vi "Main.vi"(7 "sweep rate, /min":dbl=0.2, 8 "sweep to:":dbl=4.0, 9 "sweep":T8(radio)=enum."2636a_smub") -> ()   [LabVIEW 2021] (continued)
                # "2182A 1 channel 2 measure (2182A_1_ch2)"
                n1376 = local read "2182A 1 ch2"() -> (w1691:bool)
                n1377 = property on="Figure_axis" class="Arr (strict)"() -> ("Value"=w1688:string[])  [unwired: 2 in, 2 out]
                n1378 = property on="data_caption" class="Str"() -> ("Value"=w1690:string)  [unwired: 2 in, 2 out]
                n1379 = case shown="True" w1691 {
                  tunnel: w1690 -> [w1693 w1699]
                  tunnel: [w1693 w1698] -> w1689
                  tunnel: w1688 -> [w1692 w1696]
                  tunnel: [w1692 w1694] -> w1687
                  frame False {
                    # "not measure 2182A 1 channel 2 (2182A_1_ch2)"
                  }
                  frame True {
                    w1695 = "2182A_1_ch2"
                    # "measure 2182A 1 channel 2 (2182A_1_ch2)"
                    n1380 = local read "2182A 1 addr"() -> (w1700:u8)
                    n1381 = Number To Decimal String(number=w1700) -> (decimal integer string=w1701:string)  [unwired: 1 in]
                    n1382 = GPIB Clear(3:w1701) -> ()  [unwired: 1 in, 2 out]
                    n1383 = Build Array (concatenate)(w1696, w1695) -> (w1694:string[])
                    n1384 = Concatenate Strings(w1699, w1695, "\t") -> (w1698:string)
                  }
                }
                n1385 = property on="Figure_axis" class="Arr (strict)"("Value"=w1687) -> ()  [unwired: 2 in, 2 out]
                n1386 = property on="data_caption" class="Str"("Value"=w1689) -> ()  [unwired: 2 in, 2 out]
              }
              frame #18 {
                # "2182A 2 channel 1 measure (2182A_2_ch1)"
                n1387 = local read "2182A 2 ch1"() -> (w1706:bool)
                n1388 = property on="Figure_axis" class="Arr (strict)"() -> ("Value"=w1703:string[])  [unwired: 2 in, 2 out]
                n1389 = property on="data_caption" class="Str"() -> ("Value"=w1705:string)  [unwired: 2 in, 2 out]
                n1390 = case shown="True" w1706 {
                  tunnel: w1705 -> [w1708 w1714]
                  tunnel: [w1708 w1713] -> w1704
                  tunnel: w1703 -> [w1707 w1711]
                  tunnel: [w1707 w1709] -> w1702
                  frame False {
                    # "not measure 2182A 2 channel 1 (2182A_2_ch1)"
                  }
                  frame True {
                    w1710 = "2182A_2_ch1"
                    # "measure 2182A 2 channel 1 (2182A_2_ch1)"
                    n1391 = local read "2182A 2 addr"() -> (w1715:u8)
                    n1392 = Number To Decimal String(number=w1715) -> (decimal integer string=w1716:string)  [unwired: 1 in]
                    n1393 = GPIB Clear(3:w1716) -> ()  [unwired: 1 in, 2 out]
                    n1394 = Build Array (concatenate)(w1711, w1710) -> (w1709:string[])
                    n1395 = Concatenate Strings(w1714, w1710, "\t") -> (w1713:string)
                  }
                }
                n1396 = property on="Figure_axis" class="Arr (strict)"("Value"=w1702) -> ()  [unwired: 2 in, 2 out]
                n1397 = property on="data_caption" class="Str"("Value"=w1704) -> ()  [unwired: 2 in, 2 out]
              }
              frame #19 {
                # "2182A 2 channel 2 measure (2182A_2_ch2)"
                n1398 = local read "2182A 2 ch2"() -> (w1721:bool)
                n1399 = property on="Figure_axis" class="Arr (strict)"() -> ("Value"=w1718:string[])  [unwired: 2 in, 2 out]
                n1400 = property on="data_caption" class="Str"() -> ("Value"=w1720:string)  [unwired: 2 in, 2 out]
                n1401 = case shown="True" w1721 {
                  tunnel: w1720 -> [w1723 w1729]
                  tunnel: [w1723 w1728] -> w1719
                  tunnel: w1718 -> [w1722 w1726]
                  tunnel: [w1722 w1724] -> w1717
                  frame False {
                    # "not measure 2182A 2 channel 2 (2182A_2_ch2)"
                  }
                  frame True {
                    w1725 = "2182A_2_ch2"
                    # "measure 2182A 2 channel 2 (2182A_2_ch2)"
                    n1402 = local read "2182A 2 addr"() -> (w1730:u8)
                    n1403 = Number To Decimal String(number=w1730) -> (decimal integer string=w1731:string)  [unwired: 1 in]
                    n1404 = GPIB Clear(3:w1731) -> ()  [unwired: 1 in, 2 out]
                    n1405 = Build Array (concatenate)(w1726, w1725) -> (w1724:string[])
                    n1406 = Concatenate Strings(w1729, w1725, "\t") -> (w1728:string)
                  }
                }
                n1407 = property on="Figure_axis" class="Arr (strict)"("Value"=w1717) -> ()  [unwired: 2 in, 2 out]
                n1408 = property on="data_caption" class="Str"("Value"=w1719) -> ()  [unwired: 2 in, 2 out]
              }
              frame #20 {
                # "2182A 3 channel 1 measure (2182A_3_ch1)"
                n1409 = local read "2182A 3 ch1"() -> (w1736:bool)
                n1410 = property on="Figure_axis" class="Arr (strict)"() -> ("Value"=w1733:string[])  [unwired: 2 in, 2 out]
                n1411 = property on="data_caption" class="Str"() -> ("Value"=w1735:string)  [unwired: 2 in, 2 out]
                n1412 = case shown="True" w1736 {
                  tunnel: w1735 -> [w1738 w1744]
                  tunnel: [w1738 w1743] -> w1734
                  tunnel: w1733 -> [w1737 w1741]
                  tunnel: [w1737 w1739] -> w1732
                  frame False {
                    # "not measure 2182A 3 channel 1 (2182A_3_ch1)"
                  }
                  frame True {
                    w1740 = "2182A_3_ch1"
                    # "measure 2182A 3 channel 1 (2182A_3_ch1)"
                    n1413 = local read "2182A 3 addr"() -> (w1745:u8)
                    n1414 = Number To Decimal String(number=w1745) -> (decimal integer string=w1746:string)  [unwired: 1 in]
                    n1415 = GPIB Clear(3:w1746) -> ()  [unwired: 1 in, 2 out]
                    n1416 = Build Array (concatenate)(w1741, w1740) -> (w1739:string[])
                    n1417 = Concatenate Strings(w1744, w1740, "\t") -> (w1743:string)
                  }
                }
                n1418 = property on="Figure_axis" class="Arr (strict)"("Value"=w1732) -> ()  [unwired: 2 in, 2 out]
                n1419 = property on="data_caption" class="Str"("Value"=w1734) -> ()  [unwired: 2 in, 2 out]
              }
              frame #21 {
                # "2182A 3 channel 2 measure (2182A_3_ch2)"
                n1420 = local read "2182A 3 ch2"() -> (w1751:bool)
                n1421 = property on="Figure_axis" class="Arr (strict)"() -> ("Value"=w1748:string[])  [unwired: 2 in, 2 out]
                n1422 = property on="data_caption" class="Str"() -> ("Value"=w1750:string)  [unwired: 2 in, 2 out]
                n1423 = case shown="False" w1751 {
                  tunnel: w1750 -> [w1753 w1759]
                  tunnel: [w1753 w1758] -> w1749
                  tunnel: w1748 -> [w1752 w1756]
                  tunnel: [w1752 w1754] -> w1747
                  frame False {
                    # "not measure 2182A 3 channel 2 (2182A_3_ch2)"
                  }
                  frame True {
                    w1755 = "2182A_3_ch2"
                    # "measure 2182A 3 channel 2 (2182A_3_ch2)"
                    n1424 = local read "2182A 3 addr"() -> (w1760:u8)
                    n1425 = Number To Decimal String(number=w1760) -> (decimal integer string=w1761:string)  [unwired: 1 in]
                    n1426 = GPIB Clear(3:w1761) -> ()  [unwired: 1 in, 2 out]
                    n1427 = Build Array (concatenate)(w1756, w1755) -> (w1754:string[])
                    n1428 = Concatenate Strings(w1759, w1755, "\t") -> (w1758:string)
                  }
                }
                n1429 = property on="Figure_axis" class="Arr (strict)"("Value"=w1747) -> ()  [unwired: 2 in, 2 out]
                n1430 = property on="data_caption" class="Str"("Value"=w1749) -> ()  [unwired: 2 in, 2 out]
              }
              frame #22 {
                # "2182A 4 channel 1 measure (2182A_4_ch1)"
                n1431 = local read "2182A 4 ch1"() -> (w1766:bool)
                n1432 = property on="Figure_axis" class="Arr (strict)"() -> ("Value"=w1763:string[])  [unwired: 2 in, 2 out]
                n1433 = property on="data_caption" class="Str"() -> ("Value"=w1765:string)  [unwired: 2 in, 2 out]
                n1434 = case shown="True" w1766 {
                  tunnel: w1765 -> [w1768 w1774]
                  tunnel: [w1768 w1773] -> w1764
                  tunnel: w1763 -> [w1767 w1771]
                  tunnel: [w1767 w1769] -> w1762
                  frame False {
                    # "not measure 2182A 4 channel 1 (2182A_4_ch1)"
                  }
                  frame True {
                    w1770 = "2182A_4_ch1"
                    # "measure 2182A 4 channel 1 (2182A_4_ch1)"
                    n1435 = local read "2182A 4 addr"() -> (w1775:u8)
                    n1436 = Number To Decimal String(number=w1775) -> (decimal integer string=w1776:string)  [unwired: 1 in]
                    n1437 = GPIB Clear(3:w1776) -> ()  [unwired: 1 in, 2 out]
                    n1438 = Build Array (concatenate)(w1771, w1770) -> (w1769:string[])
                    n1439 = Concatenate Strings(w1774, w1770, "\t") -> (w1773:string)
                  }
                }
                n1440 = property on="Figure_axis" class="Arr (strict)"("Value"=w1762) -> ()  [unwired: 2 in, 2 out]
                n1441 = property on="data_caption" class="Str"("Value"=w1764) -> ()  [unwired: 2 in, 2 out]
              }
              frame #23 {
                # "2182A 4 channel 2 measure (2182A_4_ch2)"
                n1442 = local read "2182A 4 ch2"() -> (w1781:bool)
                n1443 = property on="Figure_axis" class="Arr (strict)"() -> ("Value"=w1778:string[])  [unwired: 2 in, 2 out]
                n1444 = property on="data_caption" class="Str"() -> ("Value"=w1780:string)  [unwired: 2 in, 2 out]
                n1445 = case shown="True" w1781 {
                  tunnel: w1780 -> [w1783 w1789]
                  tunnel: [w1783 w1788] -> w1779
                  tunnel: w1778 -> [w1782 w1786]
                  tunnel: [w1782 w1784] -> w1777
                  frame False {
                    # "not measure 2182A 4 channel 2 (2182A_4_ch2)"
                  }
                  frame True {
                    w1785 = "2182A_4_ch2"
                    # "measure 2182A 4 channel 2 (2182A_4_ch2)"
                    n1446 = local read "2182A 4 addr"() -> (w1790:u8)
                    n1447 = Number To Decimal String(number=w1790) -> (decimal integer string=w1791:string)  [unwired: 1 in]
                    n1448 = GPIB Clear(3:w1791) -> ()  [unwired: 1 in, 2 out]
                    n1449 = Build Array (concatenate)(w1786, w1785) -> (w1784:string[])
                    n1450 = Concatenate Strings(w1789, w1785, "\t") -> (w1788:string)
                  }
                }
                n1451 = property on="Figure_axis" class="Arr (strict)"("Value"=w1777) -> ()  [unwired: 2 in, 2 out]
                n1452 = property on="data_caption" class="Str"("Value"=w1779) -> ()  [unwired: 2 in, 2 out]
              }
              frame #24 {
                # "2636A smua measure voltage (2636A_smua_v)"
                n1453 = local read "2636A smua meas v"() -> (w1796:bool)
                n1454 = property on="Figure_axis" class="Arr (strict)"() -> ("Value"=w1793:string[])  [unwired: 2 in, 2 out]
                n1455 = property on="data_caption" class="Str"() -> ("Value"=w1795:string)  [unwired: 2 in, 2 out]
                n1456 = case shown="True" w1796 {
                  tunnel: w1795 -> [w1798 w1809]
                  tunnel: [w1798 w1808] -> w1794
                  tunnel: w1793 -> [w1797 w1806]
                  tunnel: [w1797 w1804] -> w1792
                  frame False {
                    # "not measure voltage on 2636A smua (2636A_smua_v)"
                  }
                  frame True {
                    w1805 = "2614A_smua_v"
                    # "measure voltage on 2636A smua (2636A_smua_v)"
                    n1457 = local read "2614A addr"() -> (w1800:refnum<visa-resource-name>)
                    n1458 = VISA Open(VISA resource name=w1800) -> (VISA resource name=w1799:refnum<visa-resource-name>, error out=w1801:errorcluster)  [unwired: 4 in]
                    n1459 = VISA Clear(VISA resource name=w1799, error in (no error)=w1801) -> (VISA resource name out=w1803:refnum<visa-resource-name>)  [unwired: 1 out]
                    n1460 = property class="Instr"(reference=w1803, "General Settings:Timeout Value"=u32 10000) -> ()  [unwired: 1 in, 2 out]
                    n1461 = Build Array (concatenate)(w1806, w1805) -> (w1804:string[])
                    n1462 = Concatenate Strings(w1809, w1805, "\t") -> (w1808:string)
                  }
                }
                n1463 = property on="Figure_axis" class="Arr (strict)"("Value"=w1792) -> ()  [unwired: 2 in, 2 out]
                n1464 = property on="data_caption" class="Str"("Value"=w1794) -> ()  [unwired: 2 in, 2 out]
              }
              frame #25 {
                # "2636A smua measure current (2636A_smua_i)"
                n1465 = local read "2636A smua meas i"() -> (w1814:bool)
                n1466 = property on="Figure_axis" class="Arr (strict)"() -> ("Value"=w1811:string[])  [unwired: 2 in, 2 out]
                n1467 = property on="data_caption" class="Str"() -> ("Value"=w1813:string)  [unwired: 2 in, 2 out]
                n1468 = case shown="True" w1814 {
                  tunnel: w1813 -> [w1816 w1827]
                  tunnel: [w1816 w1826] -> w1812
                  tunnel: w1811 -> [w1815 w1824]
                  tunnel: [w1815 w1822] -> w1810
                  frame False {
                    # "not measure current on 2636A smua (2636A_smua_i)"
                  }
                  frame True {
                    w1823 = "2614A_smua_i"
                    # "measure current on 2636A smua (2636A_smua_i)"
                    n1469 = local read "2614A addr"() -> (w1819:refnum<visa-resource-name>)
                    n1470 = VISA Open(VISA resource name=w1819) -> (VISA resource name=w1818:refnum<visa-resource-name>, error out=w1817:errorcluster)  [unwired: 4 in]
                    n1471 = VISA Clear(VISA resource name=w1818, error in (no error)=w1817) -> (VISA resource name out=w1820:refnum<visa-resource-name>)  [unwired: 1 out]
                    n1472 = Build Array (concatenate)(w1824, w1823) -> (w1822:string[])
                    n1473 = property class="Instr"(reference=w1820, "General Settings:Timeout Value"=u32 10000) -> ()  [unwired: 1 in, 2 out]
                    n1474 = Concatenate Strings(w1827, w1823, "\t") -> (w1826:string)
                  }
                }
                n1475 = property on="Figure_axis" class="Arr (strict)"("Value"=w1810) -> ()  [unwired: 2 in, 2 out]
                n1476 = property on="data_caption" class="Str"("Value"=w1812) -> ()  [unwired: 2 in, 2 out]
              }
              frame #26 {
                # "2636A smub measure voltage (2636A_smub_v)"
                n1477 = local read "2636A smub meas v"() -> (w1832:bool)
                n1478 = property on="Figure_axis" class="Arr (strict)"() -> ("Value"=w1829:string[])  [unwired: 2 in, 2 out]
                n1479 = property on="data_caption" class="Str"() -> ("Value"=w1831:string)  [unwired: 2 in, 2 out]
                n1480 = case shown="True" w1832 {
                  tunnel: w1831 -> [w1834 w1845]
                  tunnel: [w1834 w1844] -> w1830
                  tunnel: w1829 -> [w1833 w1842]
                  tunnel: [w1833 w1840] -> w1828
                  frame False {
                    # "not measure voltage on 2636A smub (2636A_smub_v)"
                  }
                  frame True {
                    w1841 = "2614A_smub_v"
                    # "measure voltage on 2636A smub (2636A_smub_v)"
                    n1481 = local read "2614A addr"() -> (w1836:refnum<visa-resource-name>)
                    n1482 = VISA Open(VISA resource name=w1836) -> (VISA resource name=w1835:refnum<visa-resource-name>, error out=w1837:errorcluster)  [unwired: 4 in]
                    n1483 = VISA Clear(VISA resource name=w1835, error in (no error)=w1837) -> (VISA resource name out=w1838:refnum<visa-resource-name>)  [unwired: 1 out]
                    n1484 = Build Array (concatenate)(w1842, w1841) -> (w1840:string[])
                    n1485 = property class="Instr"(reference=w1838, "General Settings:Timeout Value"=u32 10000) -> ()  [unwired: 1 in, 2 out]
                    n1486 = Concatenate Strings(w1845, w1841, "\t") -> (w1844:string)
                  }
                }
                n1487 = property on="Figure_axis" class="Arr (strict)"("Value"=w1828) -> ()  [unwired: 2 in, 2 out]
                n1488 = property on="data_caption" class="Str"("Value"=w1830) -> ()  [unwired: 2 in, 2 out]
              }
              frame #27 {
                # "2636A smub measure current (2636A_smub_i)"
                n1489 = local read "2636A smub meas i"() -> (w1850:bool)
                n1490 = property on="Figure_axis" class="Arr (strict)"() -> ("Value"=w1847:string[])  [unwired: 2 in, 2 out]
                n1491 = property on="data_caption" class="Str"() -> ("Value"=w1849:string)  [unwired: 2 in, 2 out]
                n1492 = case shown="True" w1850 {
                  tunnel: w1849 -> [w1852 w1863]
                  tunnel: [w1852 w1862] -> w1848
                  tunnel: w1847 -> [w1851 w1860]
                  tunnel: [w1851 w1858] -> w1846
                  frame False {
                    # "not measure current on 2636A smub (2636A_smub_i)"
                  }
                  frame True {
                    w1859 = "2614A_smub_i"
                    # "measure current on 2614A smub (2636A_smub_i)"
                    n1493 = local read "2614A addr"() -> (w1853:refnum<visa-resource-name>)
                    n1494 = VISA Open(VISA resource name=w1853) -> (VISA resource name=w1854:refnum<visa-resource-name>, error out=w1855:errorcluster)  [unwired: 4 in]
                    n1495 = VISA Clear(VISA resource name=w1854, error in (no error)=w1855) -> (VISA resource name out=w1856:refnum<visa-resource-name>)  [unwired: 1 out]
                    n1496 = Build Array (concatenate)(w1860, w1859) -> (w1858:string[])
                    n1497 = property class="Instr"(reference=w1856, "General Settings:Timeout Value"=u32 10000) -> ()  [unwired: 1 in, 2 out]
                    n1498 = Concatenate Strings(w1863, w1859, "\t") -> (w1862:string)
                  }
                }
                n1499 = property on="Figure_axis" class="Arr (strict)"("Value"=w1846) -> ()  [unwired: 2 in, 2 out]
                n1500 = property on="data_caption" class="Str"("Value"=w1848) -> ()  [unwired: 2 in, 2 out]
              }
              frame #28 {
                # "measure time"
                n1501 = local read "measure time"() -> (w1868:bool)
                n1502 = property on="Figure_axis" class="Arr (strict)"() -> ("Value"=w1865:string[])  [unwired: 2 in, 2 out]
                n1503 = property on="data_caption" class="Str"() -> ("Value"=w1867:string)  [unwired: 2 in, 2 out]
                n1504 = case shown="True" w1868 {
                  tunnel: w1867 -> [w1870 w1876]
                  tunnel: [w1870 w1875] -> w1866
                  tunnel: w1865 -> [w1869 w1873]
                  tunnel: [w1869 w1871] -> w1864
                  frame False {
                    # "not measuring time"
                  }
                  frame True {
                    w1872 = "time"
                    # "measuring time"
                    n1505 = Build Array (concatenate)(w1873, w1872) -> (w1871:string[])
                    n1506 = Concatenate Strings(w1876, w1872, "\t") -> (w1875:string)
                  }
                }
                n1507 = property on="Figure_axis" class="Arr (strict)"("Value"=w1864) -> ()  [unwired: 2 in, 2 out]
                n1508 = property on="data_caption" class="Str"("Value"=w1866) -> ()  [unwired: 2 in, 2 out]
              }
              frame #29 {
                # "Measure magnetic field on IPS120-0"
                n1509 = local read "MagnetField"() -> (w1881:bool)
                n1510 = property on="Figure_axis" class="Arr (strict)"() -> ("Value"=w1878:string[])  [unwired: 2 in, 2 out]
                n1511 = property on="data_caption" class="Str"() -> ("Value"=w1880:string)  [unwired: 2 in, 2 out]
                n1512 = case shown="True" w1881 {
                  tunnel: w1880 -> [w1883 w1889]
                  tunnel: [w1883 w1888] -> w1879
                  tunnel: w1878 -> [w1882 w1886]
                  tunnel: [w1882 w1884] -> w1877
                  frame False {
                    # "do not Measure magnetic field on IPS120-0"
                  }
                  frame True {
                    w1885 = "MagnetField"
                    n1513 = Build Array (concatenate)(w1886, w1885) -> (w1884:string[])
                    n1514 = Concatenate Strings(w1889, w1885, "\t") -> (w1888:string)
                  }
                }
                n1515 = property on="Figure_axis" class="Arr (strict)"("Value"=w1877) -> ()  [unwired: 2 in, 2 out]
                n1516 = property on="data_caption" class="Str"("Value"=w1879) -> ()  [unwired: 2 in, 2 out]
              }
              frame #30 {
                # "Measure Magnet_T on iPS"
                n1517 = property on="Magnet_T" class="Bool (strict)"() -> ("Value"=w1890:bool)  [unwired: 2 in, 2 out]
                n1518 = property on="Figure_axis" class="Arr (strict)"() -> ("Value"=w1892:string[])  [unwired: 2 in, 2 out]
                n1519 = property on="data_caption" class="Str"() -> ("Value"=w1894:string)  [unwired: 2 in, 2 out]
                n1520 = case shown="True" w1890 {
                  tunnel: w1894 -> [w1896 w1902]
                  tunnel: [w1896 w1901] -> w1893
                  tunnel: w1892 -> [w1895 w1899]
                  tunnel: [w1895 w1897] -> w1891
                  frame False {
                    # "do not Measure magnetic field on IPS120-0"
                  }
                  frame True {
                    w1898 = "Magnet_Temp"
                    n1521 = Build Array (concatenate)(w1899, w1898) -> (w1897:string[])
                    n1522 = Concatenate Strings(w1902, w1898, "\t") -> (w1901:string)
                  }
                }
                n1523 = property on="Figure_axis" class="Arr (strict)"("Value"=w1891) -> ()  [unwired: 2 in, 2 out]
                n1524 = property on="data_caption" class="Str"("Value"=w1893) -> ()  [unwired: 2 in, 2 out]
              }
              frame #31 {
                # "Measure SH_T on iPS"
                n1525 = property on="PT1" class="Bool (strict)"() -> ("Value"=w1903:bool)  [unwired: 2 in, 2 out]
                n1526 = property on="Figure_axis" class="Arr (strict)"() -> ("Value"=w1905:string[])  [unwired: 2 in, 2 out]
                n1527 = property on="data_caption" class="Str"() -> ("Value"=w1907:string)  [unwired: 2 in, 2 out]
                n1528 = case shown="True" w1903 {
                  tunnel: w1907 -> [w1909 w1915]
                  tunnel: [w1909 w1914] -> w1906
                  tunnel: w1905 -> [w1908 w1912]
                  tunnel: [w1908 w1910] -> w1904
                  frame False {
                    # "do not Measure magnetic field on IPS120-0"
                  }
                  frame True {
                    w1911 = "PT1_Temp"
                    n1529 = Build Array (concatenate)(w1912, w1911) -> (w1910:string[])
                    n1530 = Concatenate Strings(w1915, w1911, "\t") -> (w1914:string)
                  }
                }
                n1531 = property on="Figure_axis" class="Arr (strict)"("Value"=w1904) -> ()  [unwired: 2 in, 2 out]
                n1532 = property on="data_caption" class="Str"("Value"=w1906) -> ()  [unwired: 2 in, 2 out]
              }
              frame #32 {
                # "iTC sample Temp"
                n1533 = property on="MC_RuO2" class="Bool (strict)"() -> ("Value"=w1916:bool)  [unwired: 2 in, 2 out]
                n1534 = property on="Figure_axis" class="Arr (strict)"() -> ("Value"=w1918:string[])  [unwired: 2 in, 2 out]
                n1535 = property on="data_caption" class="Str"() -> ("Value"=w1920:string)  [unwired: 2 in, 2 out]
                n1536 = case shown="True" w1916 {
                  tunnel: w1920 -> [w1922 w1928]
                  tunnel: [w1922 w1927] -> w1919
                  tunnel: w1918 -> [w1921 w1925]
                  tunnel: [w1921 w1923] -> w1917
                  frame False {
                    # "not measure 2461 voltage (2461_meas_v)"
                  }
                  frame True {
                    w1924 = "MC_RuO2_Temp"
                    n1537 = Build Array (concatenate)(w1925, w1924) -> (w1923:string[])
                    n1538 = Concatenate Strings(w1928, w1924, "\t") -> (w1927:string)
                  }
                }
                n1539 = property on="Figure_axis" class="Arr (strict)"("Value"=w1917) -> ()  [unwired: 2 in, 2 out]
                n1540 = property on="data_caption" class="Str"("Value"=w1919) -> ()  [unwired: 2 in, 2 out]
              }
              frame #33 {
                # "iTC sample Temp"
                n1541 = property on="Still" class="Bool (strict)"() -> ("Value"=w1929:bool)  [unwired: 2 in, 2 out]
                n1542 = property on="Figure_axis" class="Arr (strict)"() -> ("Value"=w1931:string[])  [unwired: 2 in, 2 out]
                n1543 = property on="data_caption" class="Str"() -> ("Value"=w1933:string)  [unwired: 2 in, 2 out]
                n1544 = case shown="True" w1929 {
                  tunnel: w1933 -> [w1935 w1941]
                  tunnel: [w1935 w1940] -> w1932
                  tunnel: w1931 -> [w1934 w1938]
                  tunnel: [w1934 w1936] -> w1930
                  frame False {
                    # "not measure 2461 voltage (2461_meas_v)"
                  }
                  frame True {
                    w1937 = "Still_Temp"
                    n1545 = Build Array (concatenate)(w1938, w1937) -> (w1936:string[])
                    n1546 = Concatenate Strings(w1941, w1937, "\t") -> (w1940:string)
                  }
                }
                n1547 = property on="Figure_axis" class="Arr (strict)"("Value"=w1930) -> ()  [unwired: 2 in, 2 out]
                n1548 = property on="data_caption" class="Str"("Value"=w1932) -> ()  [unwired: 2 in, 2 out]
              }
              frame #34 {
                # "iTC sample Temp"
                n1549 = property on="Cold_Plate" class="Bool (strict)"() -> ("Value"=w1942:bool)  [unwired: 2 in, 2 out]
                n1550 = property on="Figure_axis" class="Arr (strict)"() -> ("Value"=w1944:string[])  [unwired: 2 in, 2 out]
                n1551 = property on="data_caption" class="Str"() -> ("Value"=w1946:string)  [unwired: 2 in, 2 out]
                n1552 = case shown="True" w1942 {
                  tunnel: w1946 -> [w1948 w1954]
                  tunnel: [w1948 w1953] -> w1945
                  tunnel: w1944 -> [w1947 w1951]
                  tunnel: [w1947 w1949] -> w1943
                  frame False {
                    # "not measure 2461 voltage (2461_meas_v)"
                  }
                  frame True {
                    w1950 = "Cold_Plate_Temp"
                    n1553 = Build Array (concatenate)(w1951, w1950) -> (w1949:string[])
                    n1554 = Concatenate Strings(w1954, w1950, "\t") -> (w1953:string)
                  }
                }
                n1555 = property on="Figure_axis" class="Arr (strict)"("Value"=w1943) -> ()  [unwired: 2 in, 2 out]
                n1556 = property on="data_caption" class="Str"("Value"=w1945) -> ()  [unwired: 2 in, 2 out]
              }
              frame #35 {
                # "iTC sample Temp"
                n1557 = property on="PT2" class="Bool (strict)"() -> ("Value"=w1955:bool)  [unwired: 2 in, 2 out]
                n1558 = property on="Figure_axis" class="Arr (strict)"() -> ("Value"=w1957:string[])  [unwired: 2 in, 2 out]
                n1559 = property on="data_caption" class="Str"() -> ("Value"=w1959:string)  [unwired: 2 in, 2 out]
                n1560 = case shown="True" w1955 {
                  tunnel: w1959 -> [w1961 w1967]
                  tunnel: [w1961 w1966] -> w1958
                  tunnel: w1957 -> [w1960 w1964]
                  tunnel: [w1960 w1962] -> w1956
                  frame False {
                    # "not measure 2461 voltage (2461_meas_v)"
                  }
                  frame True {
                    w1963 = "PT2_Temp"
                    n1561 = Build Array (concatenate)(w1964, w1963) -> (w1962:string[])
                    n1562 = Concatenate Strings(w1967, w1963, "\t") -> (w1966:string)
                  }
                }
                n1563 = property on="Figure_axis" class="Arr (strict)"("Value"=w1956) -> ()  [unwired: 2 in, 2 out]
                n1564 = property on="data_caption" class="Str"("Value"=w1958) -> ()  [unwired: 2 in, 2 out]
              }
              frame #36 {
                # "iTC sample Temp"
                n1565 = property on="MC_Cernox" class="Bool (strict)"() -> ("Value"=w1968:bool)  [unwired: 2 in, 2 out]
                n1566 = property on="Figure_axis" class="Arr (strict)"() -> ("Value"=w1970:string[])  [unwired: 2 in, 2 out]
                n1567 = property on="data_caption" class="Str"() -> ("Value"=w1972:string)  [unwired: 2 in, 2 out]
                n1568 = case shown="True" w1968 {
                  tunnel: w1972 -> [w1974 w1980]
                  tunnel: [w1974 w1979] -> w1971
                  tunnel: w1970 -> [w1973 w1977]
                  tunnel: [w1973 w1975] -> w1969
                  frame False {
                    # "not measure 2461 voltage (2461_meas_v)"
                  }
                  frame True {
                    w1976 = "MC_Cernox_Temp"
                    n1569 = Build Array (concatenate)(w1977, w1976) -> (w1975:string[])
                    n1570 = Concatenate Strings(w1980, w1976, "\t") -> (w1979:string)
                  }
                }
                n1571 = property on="Figure_axis" class="Arr (strict)"("Value"=w1969) -> ()  [unwired: 2 in, 2 out]
                n1572 = property on="data_caption" class="Str"("Value"=w1971) -> ()  [unwired: 2 in, 2 out]
              }
              frame #37 {
                # "iTC sample Temp"
                n1573 = property on="2461_meas_v" class="Bool (strict)"() -> ("Value"=w1981:bool)  [unwired: 2 in, 2 out]
                n1574 = property on="Figure_axis" class="Arr (strict)"() -> ("Value"=w1983:string[])  [unwired: 2 in, 2 out]
                n1575 = property on="data_caption" class="Str"() -> ("Value"=w1985:string)  [unwired: 2 in, 2 out]
                n1576 = case shown="True" w1981 {
                  tunnel: w1985 -> [w1987 w1993]
                  tunnel: [w1987 w1992] -> w1984
                  tunnel: w1983 -> [w1986 w1990]
                  tunnel: [w1986 w1988] -> w1982
                  frame False {
                    # "not measure 2461 voltage (2461_meas_v)"
                  }
                  frame True {
                    w1989 = "2461_meas_v"
                    n1577 = Build Array (concatenate)(w1990, w1989) -> (w1988:string[])
                    n1578 = Concatenate Strings(w1993, w1989, "\t") -> (w1992:string)
                  }
                }
                n1579 = property on="Figure_axis" class="Arr (strict)"("Value"=w1982) -> ()  [unwired: 2 in, 2 out]
                n1580 = property on="data_caption" class="Str"("Value"=w1984) -> ()  [unwired: 2 in, 2 out]
              }
              frame #38 {
                # "iTC sample Temp"
                n1581 = property on="2461_meas_i" class="Bool (strict)"() -> ("Value"=w1994:bool)  [unwired: 2 in, 2 out]
                n1582 = property on="Figure_axis" class="Arr (strict)"() -> ("Value"=w1996:string[])  [unwired: 2 in, 2 out]
                n1583 = property on="data_caption" class="Str"() -> ("Value"=w1998:string)  [unwired: 2 in, 2 out]
                n1584 = case shown="True" w1994 {
                  tunnel: w1998 -> [w2000 w2006]
                  tunnel: [w2000 w2005] -> w1997
                  tunnel: w1996 -> [w1999 w2003]
                  tunnel: [w1999 w2001] -> w1995
                  frame False {
                    # "not measure 2461 voltage (2461_meas_v)"
                  }
                  frame True {
                    w2002 = "2461_meas_i"
                    n1585 = Build Array (concatenate)(w2003, w2002) -> (w2001:string[])
                    n1586 = Concatenate Strings(w2006, w2002, "\t") -> (w2005:string)
                  }
                }
                n1587 = property on="Figure_axis" class="Arr (strict)"("Value"=w1995) -> ()  [unwired: 2 in, 2 out]
                n1588 = property on="data_caption" class="Str"("Value"=w1997) -> ()  [unwired: 2 in, 2 out]
              }
              frame #39 {
                # "iTC sample Temp"
                n1589 = property on="Linetrace or Mapping?" class="Bool (strict)"() -> ("Value"=w2007:bool)  [unwired: 2 in, 2 out]
                n1590 = property on="Figure_axis" class="Arr (strict)"() -> ("Value"=w2009:string[])  [unwired: 2 in, 2 out]
                n1591 = property on="data_caption" class="Str"() -> ("Value"=w2011:string)  [unwired: 2 in, 2 out]
                n1592 = case shown="True" w2007 {
                  tunnel: w2011 -> [w2013 w2022]
                  tunnel: [w2013 w2021] -> w2010
                  tunnel: w2009 -> [w2012 w2019]
                  tunnel: [w2012 w2018] -> w2008
                  frame False {
                    # "not measure 2461 voltage (2461_meas_v)"
                  }
                  frame True {
                    n1593 = property on="step" class="RadioBtnsControl (strict)"() -> ("Value"=w2017:T5)  [unwired: 2 in, 2 out]
                    n1594 = case shown="\"V2400_1_Step\", Default" w2017 {
                      tunnel: ["V2400_1" "V2400_2" "Va" "Vb" "time" "iTC" "iPS"] -> w2015
                      frame "V2400_1_Step", Default {
                      }
                      frame "V2400_2_step" {
                      }
                      frame "2636_smua_step" {
                      }
                      frame "2636_smub_step" {
                      }
                      frame "time_step" {
                      }
                      frame "iTC_step" {
                      }
                      frame "iPS_step" {
                      }
                    }
                    n1595 = Concatenate Strings(w2015, "_Step") -> (w2014:string)
                    n1596 = Build Array (concatenate)(w2019, w2014) -> (w2018:string[])
                    n1597 = Concatenate Strings(w2022, w2014, "\t") -> (w2021:string)
                  }
                }
                n1598 = property on="Figure_axis" class="Arr (strict)"("Value"=w2008) -> ()  [unwired: 2 in, 2 out]
                n1599 = property on="data_caption" class="Str"("Value"=w2010) -> ()  [unwired: 2 in, 2 out]
              }
              frame #40 {
                # "iTC sample Temp"
                n1600 = property on="HyperLoop" class="Bool (strict)"() -> ("Value"=w2030:bool)  [unwired: 2 in, 2 out]
                n1601 = property on="Figure_axis" class="Arr (strict)"() -> ("Value"=w2032:string[])  [unwired: 2 in, 2 out]
                n1602 = property on="data_caption" class="Str"() -> ("Value"=w2034:string)  [unwired: 2 in, 2 out]
                n1603 = case shown="True" w2030 {
                  tunnel: w2034 -> [w2036 w2045]
                  tunnel: [w2036 w2044] -> w2033
                  tunnel: w2032 -> [w2035 w2042]
                  tunnel: [w2035 w2041] -> w2031
                  frame False {
                    # "not measure 2461 voltage (2461_meas_v)"
                  }
                  frame True {
                    n1604 = property on="step_hyper" class="RadioBtnsControl (strict)"() -> ("Value"=w2040:T6)  [unwired: 2 in, 2 out]
                    n1605 = case shown="\"iPS_HyperLoop\"" w2040 {
                      tunnel: ["V2400_1" "V2400_2" "Va" "Vb" "time" "iTC" "iPS"] -> w2038
                      frame "2400_1_HyperLoop", Default {
                      }
                      frame "2400_2_HyperLoop" {
                      }
                      frame "2636_smua_HyperLoop" {
                      }
                      frame "2636_smub_HyperLoop" {
                      }
                      frame "time_HyperLoop" {
                      }
                      frame "iTC_HyperLoop" {
                      }
                      frame "iPS_HyperLoop" {
                      }
                    }
                    n1606 = Concatenate Strings(w2038, "_HyperLoop") -> (w2037:string)
                    n1607 = Build Array (concatenate)(w2042, w2037) -> (w2041:string[])
                    n1608 = Concatenate Strings(w2045, w2037, "\t") -> (w2044:string)
                  }
                }
                n1609 = property on="Figure_axis" class="Arr (strict)"("Value"=w2031) -> ()  [unwired: 2 in, 2 out]
                n1610 = property on="data_caption" class="Str"("Value"=w2033) -> ()  [unwired: 2 in, 2 out]
              }
              frame #41 {
                # "iTC sample Temp"
                n1611 = property on="SuperHyper" class="Bool (strict)"() -> ("Value"=w2053:bool)  [unwired: 2 in, 2 out]
                n1612 = property on="data_caption" class="Str"() -> ("Value"=w2057:string)  [unwired: 2 in, 2 out]
                n1613 = property on="Figure_axis" class="Arr (strict)"() -> ("Value"=w2055:string[])  [unwired: 2 in, 2 out]
                n1614 = case shown="True" w2053 {
                  tunnel: w2057 -> [w2059 w2068]
                  tunnel: [w2059 w2067] -> w2056
                  tunnel: w2055 -> [w2058 w2065]
                  tunnel: [w2058 w2064] -> w2054
                  frame False {
                    # "not measure 2461 voltage (2461_meas_v)"
                  }
                  frame True {
                    n1615 = property on="step_super" class="RadioBtnsControl (strict)"() -> ("Value"=w2060:T7)  [unwired: 2 in, 2 out]
                    n1616 = case shown="\"iTC_SuperHyper\"" w2060 {
                      tunnel: ["V2400_1" "V2400_2" "Va" "Vb" "time" "iTC" "iPS"] -> w2062
                      frame "2400_1_SuperHyper", Default {
                      }
                      frame "2400_2_SuperHyper" {
                      }
                      frame "2636_smua_SuperHyper" {
                      }
                      frame "2636_smub_SuperHyper" {
                      }
                      frame "time_SuperHyper" {
                      }
                      frame "iTC_SuperHyper" {
                      }
                      frame "iPS_SuperHyper" {
                      }
                    }
                    n1617 = Concatenate Strings(w2062, "_SuperHyper") -> (w2061:string)
                    n1618 = Build Array (concatenate)(w2065, w2061) -> (w2064:string[])
                    n1619 = Concatenate Strings(w2068, w2061, "\t") -> (w2067:string)
                  }
                }
                n1620 = property on="Figure_axis" class="Arr (strict)"("Value"=w2054) -> ()  [unwired: 2 in, 2 out]
                n1621 = property on="data_caption" class="Str"("Value"=w2056) -> ()  [unwired: 2 in, 2 out]
              }
              frame #42 {
                # "MFLI_V"
                n1622 = property on="MFLI1_addr" class="Str" props=["Value"]() -> ()  [unwired: 2 in, 3 out]
                n1623 = property on="MFLI1_d0" class="Bool (strict)"() -> ("Value"=w2076:bool)  [unwired: 2 in, 2 out]
                n1624 = property on="data_caption" class="Str"() -> ("Value"=w2080:string)  [unwired: 2 in, 2 out]
                n1625 = property on="Figure_axis" class="Arr (strict)"() -> ("Value"=w2078:string[])  [unwired: 2 in, 2 out]
                n1626 = case shown="True" w2076 {
                  tunnel: w2080 -> [w2082 w2093]
                  tunnel: [w2082 w2092] -> w2079
                  tunnel: w2078 -> [w2081 w2091]
                  tunnel: [w2081 w2090] -> w2077
                  frame False {
                    # "not measure 2461 voltage (2461_meas_v)"
                  }
                  frame True {
                    w2087 = "MFLI1_d0_y"
                    w2089 = "MFLI1_d0_x"
                    w2086 = "\t"
                    w2085 = "MFLI1_d0_freq"
                    n1627 = property on="MFLI1_addr" class="Str"() -> ("Value"=w2088:string)  [unwired: 2 in, 2 out]
                    n1628 = call <instrlib>:"ziOpen.vi"("Address"=w2088) -> ("HandleOut"=w2084:T1)  [unwired: 3 in, 2 out]
                    n1629 = call <instrlib>:"ziCheckVersion.vi"("Handle In"=w2084) -> ("Handle Out"=w2083:T1)  [unwired: 12 in, 2 out]
                    n1630 = property on="HandleOut" class="Clust (strict)"("Value"=w2083) -> ()  [unwired: 2 in, 2 out]
                    n1631 = Build Array (concatenate)(w2091, w2089, w2087, w2085) -> (w2090:string[])
                    n1632 = Concatenate Strings(w2093, w2089, w2086, w2087, w2086, w2085, w2086) -> (w2092:string)
                  }
                }
                n1633 = property on="Figure_axis" class="Arr (strict)"("Value"=w2077) -> ()  [unwired: 2 in, 2 out]
                n1634 = property on="data_caption" class="Str"("Value"=w2079) -> ()  [unwired: 2 in, 2 out]
              }
              frame #43 {
                # "MFLI_V"
                n1635 = property on="MFLI2_addr" class="Str" props=["Value"]() -> ()  [unwired: 2 in, 3 out]
                n1636 = property on="MFLI2_d0" class="Bool (strict)"() -> ("Value"=w2094:bool)  [unwired: 2 in, 2 out]
                n1637 = property on="data_caption" class="Str"() -> ("Value"=w2098:string)  [unwired: 2 in, 2 out]
                n1638 = property on="Figure_axis" class="Arr (strict)"() -> ("Value"=w2096:string[])  [unwired: 2 in, 2 out]
                n1639 = case shown="True" w2094 {
                  tunnel: w2098 -> [w2100 w2111]
                  tunnel: [w2100 w2110] -> w2097
                  tunnel: w2096 -> [w2099 w2109]
                  tunnel: [w2099 w2108] -> w2095
                  frame False {
                    # "not measure 2461 voltage (2461_meas_v)"
                  }
                  frame True {
                    w2105 = "MFLI2_d0_y"
                    w2107 = "MFLI2_d0_x"
                    w2104 = "\t"
                    w2103 = "MFLI2_d0_freq"
                    n1640 = property on="MFLI2_addr" class="Str"() -> ("Value"=w2106:string)  [unwired: 2 in, 2 out]
                    n1641 = call <instrlib>:"ziOpen.vi"("Address"=w2106) -> ("HandleOut"=w2102:T1)  [unwired: 3 in, 2 out]
                    n1642 = call <instrlib>:"ziCheckVersion.vi"("Handle In"=w2102) -> ("Handle Out"=w2101:T1)  [unwired: 12 in, 2 out]
                    n1643 = property on="HandleOut 2" class="Clust (strict)"("Value"=w2101) -> ()  [unwired: 2 in, 2 out]
                    n1644 = Build Array (concatenate)(w2109, w2107, w2105, w2103) -> (w2108:string[])
                    n1645 = Concatenate Strings(w2111, w2107, w2104, w2105, w2104, w2103, w2104) -> (w2110:string)
                  }
                }
                n1646 = property on="Figure_axis" class="Arr (strict)"("Value"=w2095) -> ()  [unwired: 2 in, 2 out]
                n1647 = property on="data_caption" class="Str"("Value"=w2097) -> ()  [unwired: 2 in, 2 out]
              }
              frame #44 {
                # "MFLI_V"
                n1648 = property on="MFLI3_addr" class="Str" props=["Value"]() -> ()  [unwired: 2 in, 3 out]
                n1649 = property on="MFLI3_d0" class="Bool (strict)"() -> ("Value"=w2112:bool)  [unwired: 2 in, 2 out]
                n1650 = property on="data_caption" class="Str"() -> ("Value"=w2116:string)  [unwired: 2 in, 2 out]
                n1651 = property on="Figure_axis" class="Arr (strict)"() -> ("Value"=w2114:string[])  [unwired: 2 in, 2 out]
                n1652 = case shown="True" w2112 {
                  tunnel: w2116 -> [w2118 w2129]
                  tunnel: [w2118 w2128] -> w2115
                  tunnel: w2114 -> [w2117 w2127]
                  tunnel: [w2117 w2126] -> w2113
                  frame False {
                    # "not measure 2461 voltage (2461_meas_v)"
                  }
                  frame True {
                    w2123 = "MFLI3_d0_y"
                    w2125 = "MFLI3_d0_x"
                    w2122 = "\t"
                    w2121 = "MFLI3_d0_freq"
                    n1653 = property on="MFLI3_addr" class="Str"() -> ("Value"=w2124:string)  [unwired: 2 in, 2 out]
                    n1654 = call <instrlib>:"ziOpen.vi"("Address"=w2124) -> ("HandleOut"=w2120:T1)  [unwired: 3 in, 2 out]
                    n1655 = call <instrlib>:"ziCheckVersion.vi"("Handle In"=w2120) -> ("Handle Out"=w2119:T1)  [unwired: 12 in, 2 out]
                    n1656 = property on="HandleOut 3" class="Clust (strict)"("Value"=w2119) -> ()  [unwired: 2 in, 2 out]
                    n1657 = Build Array (concatenate)(w2127, w2125, w2123, w2121) -> (w2126:string[])
                    n1658 = Concatenate Strings(w2129, w2125, w2122, w2123, w2122, w2121, w2122) -> (w2128:string)
                  }
                }
                n1659 = property on="Figure_axis" class="Arr (strict)"("Value"=w2113) -> ()  [unwired: 2 in, 2 out]
                n1660 = property on="data_caption" class="Str"("Value"=w2115) -> ()  [unwired: 2 in, 2 out]
              }
              frame #45 {
                # "MFLI_V"
                n1661 = property on="MFLI4_addr" class="Str" props=["Value"]() -> ()  [unwired: 2 in, 3 out]
                n1662 = property on="MFLI4_d0" class="Bool (strict)"() -> ("Value"=w2130:bool)  [unwired: 2 in, 2 out]
                n1663 = property on="data_caption" class="Str"() -> ("Value"=w2134:string)  [unwired: 2 in, 2 out]
                n1664 = property on="Figure_axis" class="Arr (strict)"() -> ("Value"=w2132:string[])  [unwired: 2 in, 2 out]
                n1665 = case shown="True" w2130 {
                  tunnel: w2134 -> [w2136 w2147]
                  tunnel: [w2136 w2146] -> w2133
                  tunnel: w2132 -> [w2135 w2145]
                  tunnel: [w2135 w2144] -> w2131
                  frame False {
                    # "not measure 2461 voltage (2461_meas_v)"
                  }
                  frame True {
                    w2141 = "MFLI4_d0_y"
                    w2143 = "MFLI4_d0_x"
                    w2140 = "\t"
                    w2139 = "MFLI4_d0_freq"
                    n1666 = property on="MFLI4_addr" class="Str"() -> ("Value"=w2142:string)  [unwired: 2 in, 2 out]
                    n1667 = call <instrlib>:"ziOpen.vi"("Address"=w2142) -> ("HandleOut"=w2138:T1)  [unwired: 3 in, 2 out]
                    n1668 = call <instrlib>:"ziCheckVersion.vi"("Handle In"=w2138) -> ("Handle Out"=w2137:T1)  [unwired: 12 in, 2 out]
                    n1669 = property on="HandleOut 4" class="Clust (strict)"("Value"=w2137) -> ()  [unwired: 2 in, 2 out]
                    n1670 = Build Array (concatenate)(w2145, w2143, w2141, w2139) -> (w2144:string[])
                    n1671 = Concatenate Strings(w2147, w2143, w2140, w2141, w2140, w2139, w2140) -> (w2146:string)
                  }
                }
                n1672 = property on="Figure_axis" class="Arr (strict)"("Value"=w2131) -> ()  [unwired: 2 in, 2 out]
                n1673 = property on="data_caption" class="Str"("Value"=w2133) -> ()  [unwired: 2 in, 2 out]
              }
              frame #46 {
                # "MFLI_V"
                n1674 = property on="MFLI1_d1" class="Bool (strict)"() -> ("Value"=w2148:bool)  [unwired: 2 in, 2 out]
                n1675 = property on="data_caption" class="Str"() -> ("Value"=w2152:string)  [unwired: 2 in, 2 out]
                n1676 = property on="Figure_axis" class="Arr (strict)"() -> ("Value"=w2150:string[])  [unwired: 2 in, 2 out]
                n1677 = case shown="True" w2148 {
                  tunnel: w2152 -> [w2154 w2162]
                  tunnel: [w2154 w2161] -> w2151
                  tunnel: w2150 -> [w2153 w2160]
                  tunnel: [w2153 w2159] -> w2149
                  frame False {
                    # "not measure 2461 voltage (2461_meas_v)"
                  }
                  frame True {
                    w2157 = "MFLI1_d1_y"
                    w2158 = "MFLI1_d1_x"
                    w2156 = "\t"
                    w2155 = "MFLI1_d1_freq"
                    n1678 = Build Array (concatenate)(w2160, w2158, w2157, w2155) -> (w2159:string[])
                    n1679 = Concatenate Strings(w2162, w2158, w2156, w2157, w2156, w2155, w2156) -> (w2161:string)
                  }
                }
                n1680 = property on="Figure_axis" class="Arr (strict)"("Value"=w2149) -> ()  [unwired: 2 in, 2 out]
                n1681 = property on="data_caption" class="Str"("Value"=w2151) -> ()  [unwired: 2 in, 2 out]
              }
              frame #47 {
                # "MFLI_V"
                n1682 = property on="MFLI2_d1" class="Bool (strict)"() -> ("Value"=w2163:bool)  [unwired: 2 in, 2 out]
                n1683 = property on="data_caption" class="Str"() -> ("Value"=w2167:string)  [unwired: 2 in, 2 out]
                n1684 = property on="Figure_axis" class="Arr (strict)"() -> ("Value"=w2165:string[])  [unwired: 2 in, 2 out]
                n1685 = case shown="True" w2163 {
                  tunnel: w2167 -> [w2169 w2177]
                  tunnel: [w2169 w2176] -> w2166
                  tunnel: w2165 -> [w2168 w2175]
                  tunnel: [w2168 w2174] -> w2164
                  frame False {
                    # "not measure 2461 voltage (2461_meas_v)"
                  }
                  frame True {
                    w2172 = "MFLI1_d1_y"
                    w2173 = "MFLI2_d1_x"
                    w2171 = "\t"
                    w2170 = "MFLI2_d1_freq"
                    n1686 = Build Array (concatenate)(w2175, w2173, w2172, w2170) -> (w2174:string[])
                    n1687 = Concatenate Strings(w2177, w2173, w2171, w2172, w2171, w2170, w2171) -> (w2176:string)
                  }
                }
                n1688 = property on="Figure_axis" class="Arr (strict)"("Value"=w2164) -> ()  [unwired: 2 in, 2 out]
                n1689 = property on="data_caption" class="Str"("Value"=w2166) -> ()  [unwired: 2 in, 2 out]
              }
              frame #48 {
                # "MFLI_V"
                n1690 = property on="MFLI3_d1" class="Bool (strict)"() -> ("Value"=w2178:bool)  [unwired: 2 in, 2 out]
                n1691 = property on="data_caption" class="Str"() -> ("Value"=w2182:string)  [unwired: 2 in, 2 out]
                n1692 = property on="Figure_axis" class="Arr (strict)"() -> ("Value"=w2180:string[])  [unwired: 2 in, 2 out]
                n1693 = case shown="True" w2178 {
                  tunnel: w2182 -> [w2184 w2192]
                  tunnel: [w2184 w2191] -> w2181
                  tunnel: w2180 -> [w2183 w2190]
                  tunnel: [w2183 w2189] -> w2179
                  frame False {
                    # "not measure 2461 voltage (2461_meas_v)"
                  }
                  frame True {
                    w2187 = "MFLI3_d1_y"
                    w2188 = "MFLI3_d1_x"
                    w2186 = "\t"
                    w2185 = "MFLI3_d1_freq"
                    n1694 = Build Array (concatenate)(w2190, w2188, w2187, w2185) -> (w2189:string[])
                    n1695 = Concatenate Strings(w2192, w2188, w2186, w2187, w2186, w2185, w2186) -> (w2191:string)
                  }
                }
                n1696 = property on="Figure_axis" class="Arr (strict)"("Value"=w2179) -> ()  [unwired: 2 in, 2 out]
                n1697 = property on="data_caption" class="Str"("Value"=w2181) -> ()  [unwired: 2 in, 2 out]
              }
              frame #49 {
                # "MFLI_V"
                n1698 = property on="MFLI4_d1" class="Bool (strict)"() -> ("Value"=w2193:bool)  [unwired: 2 in, 2 out]
                n1699 = property on="data_caption" class="Str"() -> ("Value"=w2197:string)  [unwired: 2 in, 2 out]
                n1700 = property on="Figure_axis" class="Arr (strict)"() -> ("Value"=w2195:string[])  [unwired: 2 in, 2 out]
                n1701 = case shown="True" w2193 {
                  tunnel: w2197 -> [w2199 w2207]
                  tunnel: [w2199 w2206] -> w2196
                  tunnel: w2195 -> [w2198 w2205]
                  tunnel: [w2198 w2204] -> w2194
                  frame False {
                    # "not measure 2461 voltage (2461_meas_v)"
                  }
                  frame True {
                    w2202 = "MFLI4_d1_y"
                    w2203 = "MFLI4_d1_x"
                    w2201 = "\t"
                    w2200 = "MFLI4_d1_freq"
                    n1702 = Build Array (concatenate)(w2205, w2203, w2202, w2200) -> (w2204:string[])
                    n1703 = Concatenate Strings(w2207, w2203, w2201, w2202, w2201, w2200, w2201) -> (w2206:string)
                  }
                }
                n1704 = property on="Figure_axis" class="Arr (strict)"("Value"=w2194) -> ()  [unwired: 2 in, 2 out]
                n1705 = property on="data_caption" class="Str"("Value"=w2196) -> ()  [unwired: 2 in, 2 out]
              }
              frame #50 {
                # "MFLI_V"
                n1706 = property on="MFLI1_d2" class="Bool (strict)"() -> ("Value"=w2208:bool)  [unwired: 2 in, 2 out]
                n1707 = property on="data_caption" class="Str"() -> ("Value"=w2212:string)  [unwired: 2 in, 2 out]
                n1708 = property on="Figure_axis" class="Arr (strict)"() -> ("Value"=w2210:string[])  [unwired: 2 in, 2 out]
                n1709 = case shown="True" w2208 {
                  tunnel: w2212 -> [w2214 w2222]
                  tunnel: [w2214 w2221] -> w2211
                  tunnel: w2210 -> [w2213 w2220]
                  tunnel: [w2213 w2219] -> w2209
                  frame False {
                    # "not measure 2461 voltage (2461_meas_v)"
                  }
                  frame True {
                    w2217 = "MFLI1_d2_y"
                    w2218 = "MFLI1_d2_x"
                    w2216 = "\t"
                    w2215 = "MFLI1_d2_freq"
                    n1710 = Build Array (concatenate)(w2220, w2218, w2217, w2215) -> (w2219:string[])
                    n1711 = Concatenate Strings(w2222, w2218, w2216, w2217, w2216, w2215, w2216) -> (w2221:string)
                  }
                }
                n1712 = property on="Figure_axis" class="Arr (strict)"("Value"=w2209) -> ()  [unwired: 2 in, 2 out]
                n1713 = property on="data_caption" class="Str"("Value"=w2211) -> ()  [unwired: 2 in, 2 out]
              }
              frame #51 {
                # "MFLI_V"
                n1714 = property on="MFLI2_d2" class="Bool (strict)"() -> ("Value"=w2223:bool)  [unwired: 2 in, 2 out]
                n1715 = property on="data_caption" class="Str"() -> ("Value"=w2227:string)  [unwired: 2 in, 2 out]
                n1716 = property on="Figure_axis" class="Arr (strict)"() -> ("Value"=w2225:string[])  [unwired: 2 in, 2 out]
                n1717 = case shown="True" w2223 {
                  tunnel: w2227 -> [w2229 w2237]
                  tunnel: [w2229 w2236] -> w2226
                  tunnel: w2225 -> [w2228 w2235]
                  tunnel: [w2228 w2234] -> w2224
                  frame False {
                    # "not measure 2461 voltage (2461_meas_v)"
                  }
                  frame True {
                    w2232 = "MFLI2_d2_y"
                    w2233 = "MFLI2_d2_x"
                    w2231 = "\t"
                    w2230 = "MFLI2_d2_freq"
                    n1718 = Build Array (concatenate)(w2235, w2233, w2232, w2230) -> (w2234:string[])
                    n1719 = Concatenate Strings(w2237, w2233, w2231, w2232, w2231, w2230, w2231) -> (w2236:string)
                  }
                }
                n1720 = property on="Figure_axis" class="Arr (strict)"("Value"=w2224) -> ()  [unwired: 2 in, 2 out]
                n1721 = property on="data_caption" class="Str"("Value"=w2226) -> ()  [unwired: 2 in, 2 out]
              }
              frame #52 {
                # "MFLI_V"
                n1722 = property on="MFLI3_d2" class="Bool (strict)"() -> ("Value"=w2238:bool)  [unwired: 2 in, 2 out]
                n1723 = property on="data_caption" class="Str"() -> ("Value"=w2242:string)  [unwired: 2 in, 2 out]
                n1724 = property on="Figure_axis" class="Arr (strict)"() -> ("Value"=w2240:string[])  [unwired: 2 in, 2 out]
                n1725 = case shown="True" w2238 {
                  tunnel: w2242 -> [w2244 w2252]
                  tunnel: [w2244 w2251] -> w2241
                  tunnel: w2240 -> [w2243 w2250]
                  tunnel: [w2243 w2249] -> w2239
                  frame False {
                    # "not measure 2461 voltage (2461_meas_v)"
                  }
                  frame True {
                    w2247 = "MFLI3_d2_y"
                    w2248 = "MFLI3_d2_x"
                    w2246 = "\t"
                    w2245 = "MFLI3_d2_freq"
                    n1726 = Build Array (concatenate)(w2250, w2248, w2247, w2245) -> (w2249:string[])
                    n1727 = Concatenate Strings(w2252, w2248, w2246, w2247, w2246, w2245, w2246) -> (w2251:string)
                  }
                }
                n1728 = property on="Figure_axis" class="Arr (strict)"("Value"=w2239) -> ()  [unwired: 2 in, 2 out]
                n1729 = property on="data_caption" class="Str"("Value"=w2241) -> ()  [unwired: 2 in, 2 out]
              }
              frame #53 {
                # "MFLI_V"
                n1730 = property on="MFLI4_d2" class="Bool (strict)"() -> ("Value"=w2253:bool)  [unwired: 2 in, 2 out]
                n1731 = property on="data_caption" class="Str"() -> ("Value"=w2257:string)  [unwired: 2 in, 2 out]
                n1732 = property on="Figure_axis" class="Arr (strict)"() -> ("Value"=w2255:string[])  [unwired: 2 in, 2 out]
                n1733 = case shown="True" w2253 {
                  tunnel: w2257 -> [w2259 w2267]
                  tunnel: [w2259 w2266] -> w2256
                  tunnel: w2255 -> [w2258 w2265]
                  tunnel: [w2258 w2264] -> w2254
                  frame False {
                    # "not measure 2461 voltage (2461_meas_v)"
                  }
                  frame True {
                    w2262 = "MFLI4_d2_y"
                    w2263 = "MFLI4_d2_x"
                    w2261 = "\t"
                    w2260 = "MFLI4_d2_freq"
                    n1734 = Build Array (concatenate)(w2265, w2263, w2262, w2260) -> (w2264:string[])
                    n1735 = Concatenate Strings(w2267, w2263, w2261, w2262, w2261, w2260, w2261) -> (w2266:string)
                  }
                }
                n1736 = property on="Figure_axis" class="Arr (strict)"("Value"=w2254) -> ()  [unwired: 2 in, 2 out]
                n1737 = property on="data_caption" class="Str"("Value"=w2256) -> ()  [unwired: 2 in, 2 out]
              }
              frame #54 {
                # "MFLI_V"
